vi "Write_Results_file.vi"(0 "Experiment start time":dbl, 1 "Experiment End time":dbl, 3 "Setup filename":string) -> ()   [LabVIEW 2011]
uses:
  Controls/Post_Process.ctl
  Globals/Meas_global.vi
  Globals/Trav_pos_global.vi
  Globals/Dynamic_call_global.ph.vi
panel:
  out "x-y":u32
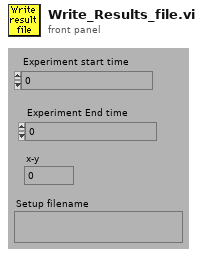
[diagram p1: front panel]
types:
  T1 = typedef "Post_Process.ctl" = enum16{"Take New Data", "Post Process Raw Data File"}
  T2 = enum16{"Save no data", "Save data in new files", "Save data in existing files"}
  T3 = typedef "Analysis_info_cluster.ctl" = cluster{"Colour":u32, "Inst type":T4, "Inst name":string, "Symbol":string, "Code name":string, "Extra Info":string, "Inst Array":T5, "Index":i32, "Voltage Index":i32, "Extra Titles":string[], "Extra Values":string[], "Eng Values":dbl[], "Time (ms)":dbl[], "Voltage":dbl[], "U":dbl, "u^2":dbl, "u^3":dbl, "u^4":dbl, "Skew_u":dbl, "Kurt_u":dbl, "Sd Error in Mean":dbl, "% u'/U":dbl, "X":dbl, "Y":dbl, "Z":dbl, "Spectra":T6, "Autocorrelation":T6, "Timescale integral to 25%":dbl, "Sd Error in Variance":dbl, "Calib File":path, "Calib Constants":dbl[], "Histogram":T6, "Output Position":bool, "Full Stats":bool, "Weighting":dbl[]}
  T4 = typedef "Inst_type.ctl" = enum16{"Propeller anemometer", "Raw voltage", "Pressure Transducer", "Pitot-static tube", "Preston tube", "Hot wire", "Cross wire 1", "Cross wire 2", "Generic Linear", "Generic Polynomial", "Generic BackPoly", "Fast FID", "Thermocouple", "Cold wire", "Pulsed Wire", "LDA Vel", "LDA Tran time", "LDA Arr time"}
  T5 = typedef "Instrument_Array.ctl" = enum16{"PWA", "LDA", "Analogue"}
  T6 = typedef "XY_Plot_Cluster.ctl" = cluster{"First Name":string, "Second Name":string, "X axis name":string, "Y axis name":string, "X array":dbl[], "Y array":dbl[]}
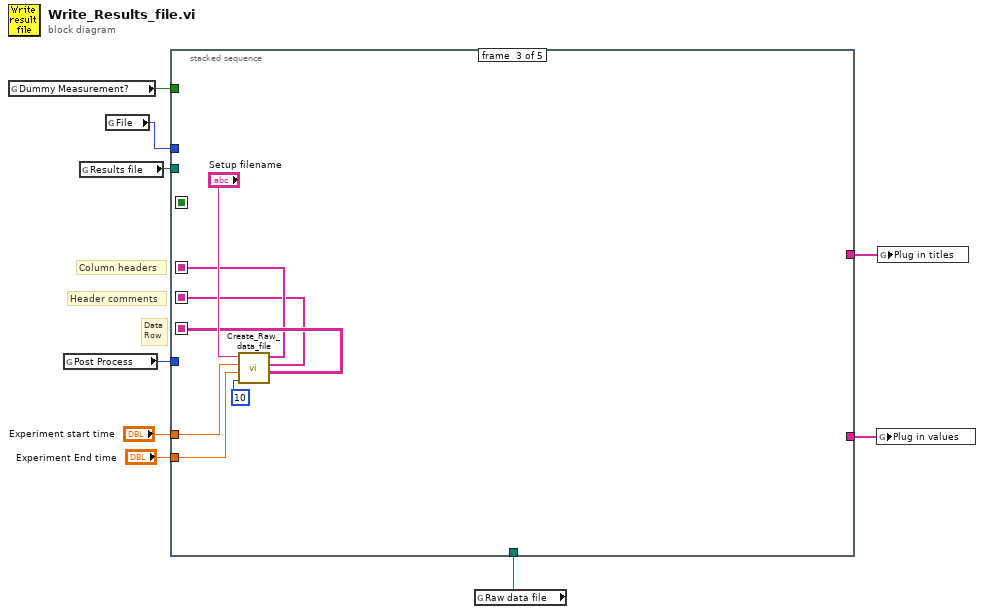
[diagram p0: block diagram]
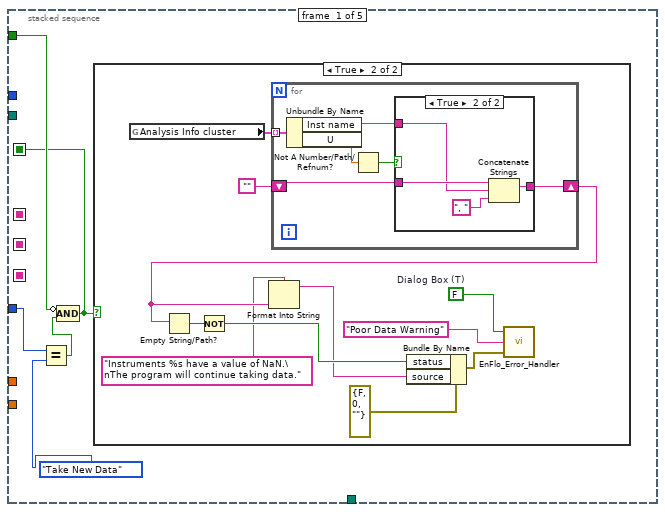
[diagram p2: hidden frame]
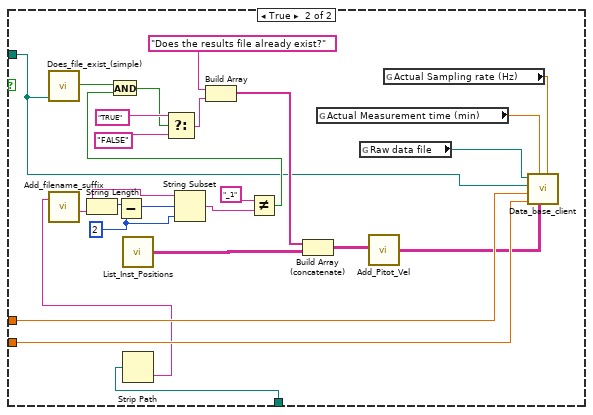
[diagram p6: hidden frame]
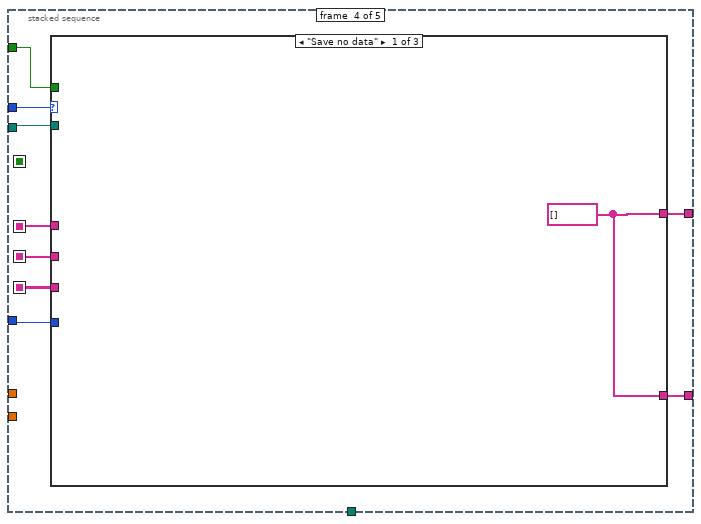
[diagram p7: hidden frame]
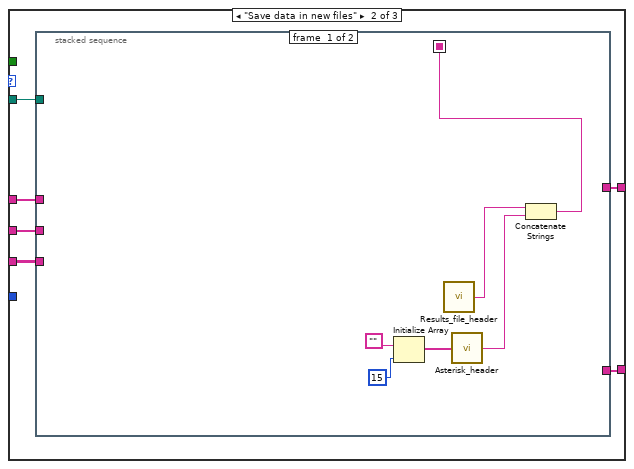
[diagram p8: hidden frame]
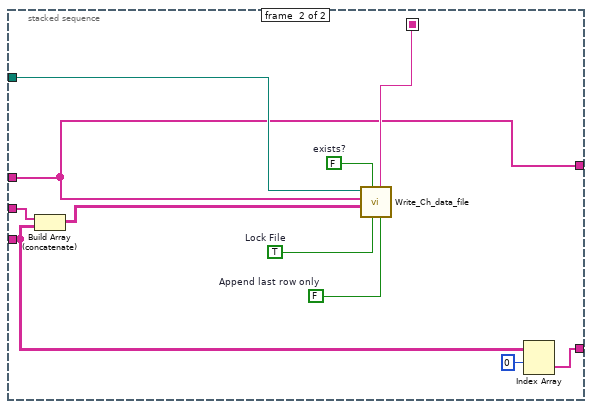
[diagram p9: hidden frame]
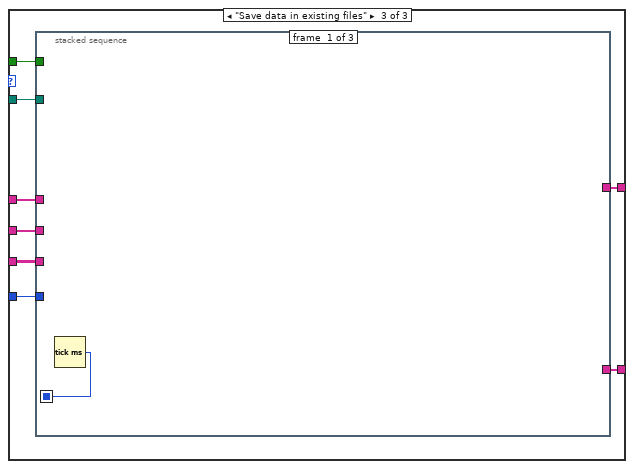
[diagram p10: hidden frame]
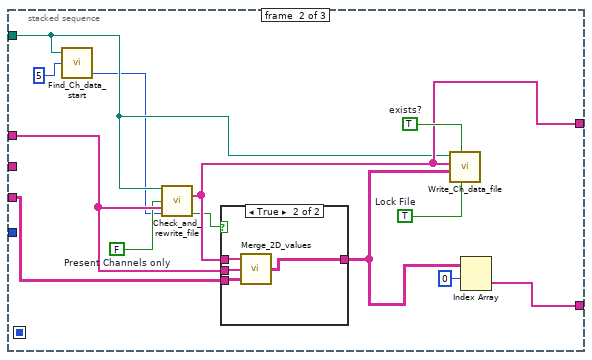
[diagram p11: hidden frame]
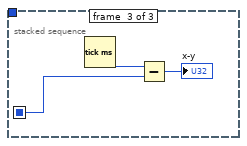
[diagram p13: hidden frame]
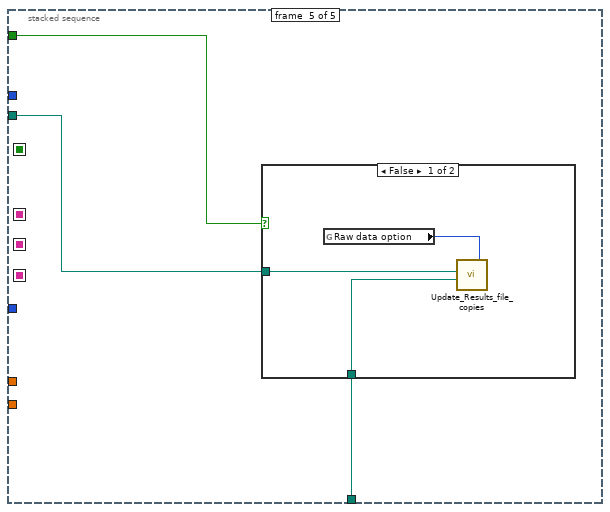
[diagram p14: hidden frame]
diagram:
  # "Data\nRow"
  # "Header comments"
  # "Column headers"
  n1 = global read "Trav_pos_global.vi" "Dummy Measurement?"() -> (w1:bool)
  n2 = global read "Meas_global.vi" "Post Process"() -> (w5:T1)
  n3 = global read "Meas_global.vi" "Results file"() -> (w2:path)
  n4 = global read "Meas_global.vi" "File"() -> (w9:T2)
  n5 = global read "Meas_global.vi" "Raw data file"() -> (w8:path)
  n6 = stacked-sequence {
    seq-local: [_ _ w68 _ _] -> [_ _ _ w81 _]
    seq-local: [_ _ w69 _ _] -> [_ _ _ w80 _]
    seq-local: [_ _ w67 _ _] -> [_ _ _ w79 _]
    seq-local: [w10 _ _ _ _] -> [_ w38 _ _ _]
    tunnel: w9 -> [_ _ _ w82 _]
    tunnel: w8 -> [_ w37 _ _ w139]
    tunnel: "Experiment start time" -> [_ w41 w73 _ _]
    tunnel: "Experiment End time" -> [_ w40 w72 _ _]
    tunnel: w5 -> [w13 _ _ w78 _]
    tunnel: [_ _ _ w77 _] -> w4
    tunnel: [_ _ _ w76 _] -> w3
    tunnel: w2 -> [_ w39 _ w75 w138]
    tunnel: w1 -> [w11 _ _ w74 w137]
    frame #0 {
      n7 = Equal?(x=w13, y=Post_Process."Take New Data" ("Post Process")) -> (x = y?=w12:bool)
      n8 = Compound Arithmetic op=AND(invert w11, w12) -> (w10:bool)
      n9 = case shown="True" w10 {
        frame False {
        }
        frame True {
          w22 = FALSE  # Dialog Box (T)
          n10 = global read "Meas_global.vi" "Analysis Info cluster"() -> (w25:T3[])
          n11 = for {
            tunnel: w25 -> [w31] mode=indexing
            shift-right: [w26] -> w17
            shift-left: "" -> [w28]
            n12 = Unbundle By Name(w31) -> ("Inst name"=w27:string, "U"=w30:dbl)
            n13 = Not A Number/Path/Refnum?(number/path/refnum=w30) -> (NaN/Path/Refnum?=w29:bool)
            n14 = case shown="True" w29 {
              tunnel: w28 -> [w32 w36]
              tunnel: w27 -> [_ w35]
              tunnel: [w32 w33] -> w26
              frame False {
              }
              frame True {
                n15 = Concatenate Strings(w36, w35, ", " ("Substring")) -> (w33:string)
              }
            }
          }
          n16 = Empty String/Path?(string/path=w17) -> (empty?=w19:bool)
          n17 = Not(x=w19) -> (.not. x?=w18:bool)
          n18 = Format Into String(format string="Instruments %s have a value of NaN.\nThe program will continue taking data." ("Format String"), w17) -> (resulting string=w15:string)  [unwired: 2 in, 1 out]
          n19 = Bundle By Name(cluster=errorcluster {"status"=FALSE, "code"=0, "source"=""} ("error in (no error)"), "status"=w18, "source"=w15) -> (w20:errorcluster)
          n20 = call "EnFlo_Error_Handler.vi"("error in (no error)"=w20, "Error Type"="Poor Data Warning", "Dialog Box (T)"=w22) -> ()  [unwired: 3 out]
        }
      }
    }
    frame #1 {
      n21 = case shown="False" w38 {
        tunnel: w41 -> [_ w64]
        tunnel: w40 -> [_ w63]
        tunnel: w39 -> [_ w43]
        tunnel: w37 -> [_ w54]
        frame False {
        }
        frame True {
          w49 = 2 ("y")
          n22 = call "Does_file_exist_(simple).vi"("Pathname"=w43) -> ("exists?"=w46:bool)
          n23 = call "List_Inst_Positions.vi"() -> ("Position Info"=w58:string[][])  [unwired: 1 in]
          n24 = Strip Path(path=w54) -> (name=w53:string)  [unwired: 1 out]
          n25 = call "Add_filename_suffix.vi"("Filename"=w53) -> ("Base name"=w52:string)  [unwired: 1 in, 3 out]
          n26 = String Length(string=w52) -> (length=w51:i32)
          n27 = Subtract(x=w51, y=w49) -> (x-y=w50:i32)
          n28 = String Subset(string=w52, offset (0)=w50, length (rest)=w49) -> (substring=w48:string)
          n29 = Not Equal?(x="_1", y=w48) -> (x != y?=w45:bool)
          n30 = And(x=w46, y=w45) -> (x .and. y?=w44:bool)
          n31 = Select(t="TRUE", s=w44, f="FALSE") -> (s? t:f=w61:string)
          n32 = Build Array("Does the results file already exist?", w61) -> (w57:string[])
          n33 = Build Array (concatenate)(w57, w58) -> (w56:string[][])
          n34 = global read "Meas_global.vi" "Actual Measurement time (min)"() -> (w66:dbl)
          n35 = global read "Meas_global.vi" "Raw data file"() -> (w42:path)
          n36 = call "Add_Pitot_Vel.vi"("Channels from Client In"=w56) -> ("Channels from Client Out"=w55:string[][])
          n37 = global read "Meas_global.vi" "Actual Sampling rate (Hz)"() -> (w65:dbl)
          n38 = call "Data_base_client.vi"("Average Sampling freq"=w65, "Channels from Client"=w55, "Average Meas Time (min)"=w66, "End time"=w63, "Start time"=w64, "Results File Pathname"=w43, "Raw Data Pathname"=w42) -> ()  [unwired: 4 out]
        }
      }
    }
    frame #2 {
      n39 = call "Create_Raw_data_file.vi"("No of averages"=10, "End time"=w72, "Start time"=w73, "Setup filename"="Setup filename") -> ("Values"=w69:string[][], "Header Comments"=w67:string[], "Column headers"=w68:string[])  [unwired: 1 out]
    }
    frame #3 {
      n40 = case shown="\"Save no data\"" w82 {
        tunnel: w81 -> [_ w89 w114]
        tunnel: w80 -> [_ w88 w113]
        tunnel: w79 -> [_ w87 w112]
        tunnel: w75 -> [_ w86 w111]
        tunnel: w78 -> [_ _ w110]
        tunnel: [w83 w84 w109] -> w77
        tunnel: [w83 w85 w108] -> w76
        tunnel: w74 -> [_ _ w107]
        frame "Save no data" {
          w83 = string[] [] ("Merged Channels")
        }
        frame "Save data in new files" {
          n41 = stacked-sequence {
            seq-local: [w90 _] -> [_ w103]
            tunnel: w89 -> [_ w99]
            tunnel: w88 -> [_ w97]
            tunnel: w87 -> [_ w105]
            tunnel: w86 -> [_ w101]
            tunnel: [_ w99] -> w85
            tunnel: [_ w96] -> w84
            frame #0 {
              n42 = Initialize Array("", 15) -> (w94:string[])
              n43 = call "Results_file_header.vi"() -> ("Header"=w95:string)
              n44 = call "Asterisk_header.vi"("Channel names"=w94) -> ("Header string"=w91:string)
              n45 = Concatenate Strings(w95, w91) -> (w90:string)
            }
            frame #1 {
              w100 = TRUE  # Lock File
              w102 = FALSE  # Append last row only
              w106 = FALSE  # exists?
              n46 = Build Array (concatenate)(w105, w97) -> (w104:string[][])
              n47 = call "Write_Ch_data_file.vi"("Append last row only"=w102, "Header string"=w103, "Lock File"=w100, "exists?"=w106, "Channel Values"=w104, "Channel names"=w99, "Filename"=w101) -> ()  [unwired: 1 in, 4 out]
              n48 = Index Array(array=w97, index (row)=0) -> (element=w96:string[])  [unwired: 1 in]
            }
          }
        }
        frame "Save data in existing files" {
          n49 = stacked-sequence {
            seq-local: [w115 _ _] -> [_ _ w135]
            tunnel: w114 -> [_ w126 _]
            tunnel: w113 -> [_ w127 _]
            tunnel: w112 -> [_ _ _]
            tunnel: w111 -> [_ w122 _]
            tunnel: w110 -> [_ _ _]
            tunnel: [_ w116 _] -> w109
            tunnel: [_ w124 _] -> w108
            tunnel: w107 -> [_ _ _]
            frame #0 {
              n50 = Tick Count (ms)() -> (millisecond timer value=w115:u32)
            }
            frame #1 {
              w123 = FALSE  # Present Channels only
              w125 = TRUE  # Lock File
              w128 = TRUE  # exists?
              n51 = call "Find_Ch_data_start.vi"("Approx No Of Columns"=5, "Filename"=w122) -> ("Start of read offset output"=w120:i32)  [unwired: 1 in, 2 out]
              n52 = call "Check_and_rewrite_file.vi"("Filename"=w122, "Present Channels only"=w123, "Present Channels"=w126, "Start of read offset (chars.: 0)"=w120) -> ("Merged Channels"=w124:string[], "Merged?"=w119:bool)  [unwired: 10 out]
              n53 = case shown="True" w119 {
                tunnel: w127 -> [w129 w131]
                tunnel: w126 -> [_ w132]
                tunnel: [w129 w130] -> w117
                tunnel: w124 -> [_ w133]
                frame False {
                }
                frame True {
                  n54 = call "Merge_2D_values.vi"("Values In"=w131, "Present Channels"=w132, "Desired Channels"=w133) -> ("Values Out"=w130:string[][])
                }
              }
              n55 = call "Write_Ch_data_file.vi"("Lock File"=w125, "exists?"=w128, "Channel Values"=w117, "Channel names"=w124, "Filename"=w122) -> ()  [unwired: 3 in, 4 out]
              n56 = Index Array(array=w117, index (row)=0) -> (element=w116:string[])  [unwired: 1 in]
            }
            frame #2 {
              n57 = Tick Count (ms)() -> (millisecond timer value=w136:u32)
              n58 = Subtract(x=w136, y=w135) -> (x-y=→"x-y":u32)
            }
          }
        }
      }
    }
    frame #4 {
      n59 = case shown="False" w137 {
        tunnel: w139 -> [w142 _]
        tunnel: w138 -> [w140 _]
        frame False {
          n60 = global read "Meas_global.vi" "Raw data option"() -> (w141:enum16{"Save raw data", "Raw data not saved"})
          n61 = call "Update_Results_file_copies.vi"("Raw data option"=w141, "Raw data file"=w142, "Results file"=w140) -> ()  [unwired: 4 out]
        }
        frame True {
        }
      }
    }
  }
  n62 = global write "Dynamic_call_global.ph.vi" "Plug in values"(w4) -> ()
  n63 = global write "Dynamic_call_global.ph.vi" "Plug in titles"(w3) -> ()
